vi "process.vi"(8 "error in":errorcluster, 9 "result allocation":T1, 10 "parameters":T1, 11 "module in":refnum<class "Profibus Module runtime.lvclass">) -> (0 "error out":errorcluster, 1 "results":T1, 2 "parameter allocation":T1, 3 "module out":refnum<class "Profibus Module runtime.lvclass">)   [LabVIEW 2013, in "Profibus Module runtime.lvclass"]
doc: "Provides an interface for information processing by a module at runtime. While this interface performs no operations, a child should provide an override which may process data in any manner necessary."
uses:
  Profibus Module runtime.lvclass
  <vilib>/NI/Tag Bus/table/data table.ctl
  Profibus Module runtime.lvclass/Profibus Module runtime.ctl
  dynamic profibus/dynamic profibus.lvlib
  <vilib>/NI/Tag Bus/table/data table.lvlib
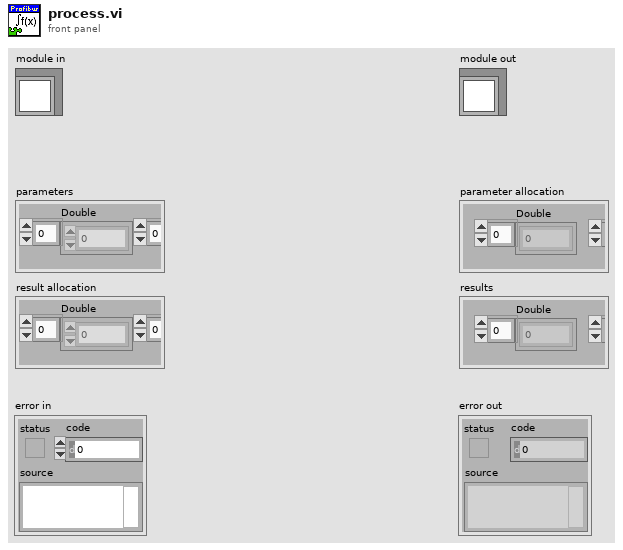
[diagram p1: front panel]
types:
  T1 = typedef "tag bus.lvlib/data table.lvlib/data table.ctl" = cluster{"Double":dbl[], "Single":sgl[], "I64":i64[], "I32":i32[], "I16":i16[], "I8":i8[], "U64":u64[], "U32":u32[], "U16":u16[], "U8":u8[], "Boolean":bool[], "String":string[], "Array of Double":cluster{"DBL Array":dbl[]}[], "Array of Single":cluster{"SGL Array":sgl[]}[], "Array of I64":cluster{"I64 Array":i64[]}[], "Array of I32":cluster{"I32 Array":i32[]}[], "Array of I16":cluster{"I16 Array":i16[]}[], "Array of I8":cluster{"I8 Array":i8[]}[], "Array of U64":cluster{"U64 Array":u64[]}[], "Array of U32":cluster{"U32 Array":u32[]}[], "Array of U16":cluster{"U16 Array":u16[]}[], "Array of U8":cluster{"U8 Array":u8[]}[], "Array of Boolean":cluster{"Boolean Array":bool[]}[], "Array of String":cluster{"String Array":string[]}[]}
  T2 = typedef "dynamic profibus.lvlib/CS_cRIO-PB_DP-Master_FPGA-Reference.ctl" = refnum<k20>
  T3 = enum16{"Start/Stop DP-Master", "Get Input Data", "Set Output Data", "Get Output Data", "Get Diagnostic Data", "Read/Write Data", "Read Diagnostic Data", "Get DPV1 Data", "Set DPV1 Data", "Read/Write DPV1 Data"}
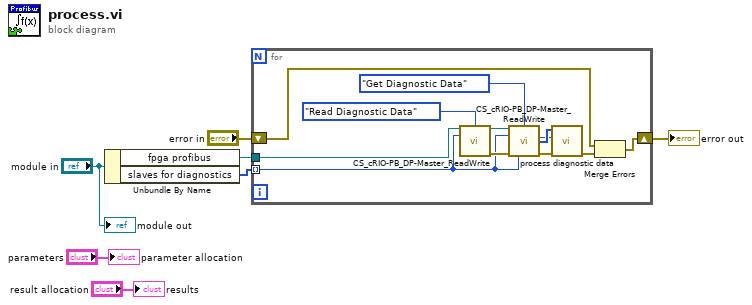
[diagram p0: block diagram]
diagram:
  n1 = Unbundle By Name("module in") -> ("fpga profibus"=w4:T2, "slaves for diagnostics"=w2:i8[])
  n2 = for {
    tunnel: w4 -> [w14]
    tunnel: w2 -> [w8] mode=indexing
    shift-right: [w12] -> w1
    shift-left: "error in" -> [w13]
    n3 = call "CS_cRIO-PB_DP-Master_ReadWrite.vi"("FPGA VI Reference"=w14, "Mode"=T3."Read Diagnostic Data", "Slave"=w8) -> ("FPGA VI Reference out"=w16:T2, "Error out"=w17:errorcluster)  [unwired: 9 in, 2 out]
    n4 = call "CS_cRIO-PB_DP-Master_ReadWrite.vi"("FPGA VI Reference"=w16, "Mode"=T3."Get Diagnostic Data", "Slave"=w8, "Error"=w17) -> ("Data out"=w9:u8[], "Error out"=w10:errorcluster)  [unwired: 8 in, 2 out]
    n5 = call "process diagnostic data.vi"("error in"=w10, "expected slave"=w8, "diagnostic bytes"=w9) -> ("error out"=w11:errorcluster)  [unwired: 8 in]
    n6 = Merge Errors(w13, w11) -> (w12:errorcluster)
  }
  "error out" <- w1
  "module out" <- "module in"
  "results" <- "result allocation"
  "parameter allocation" <- "parameters"
